vi "fpga_RefCH Process (50Hz).vi"(0 "data in <?24.1>":fxp<+/-,24,1>, 5 "Channel number":u8, 7 "Reference index":u8, 9 "input data valid":bool, 12 "ready for output":bool) -> (4 "Filtered Ref data":fxp<+/-,24,3> format="%.22g", 10 "output valid":bool, 15 "Timed Out":bool)   [LabVIEW 2011, in "NI_EP_Resample_FPGA.lvlib"]
uses:
  <vilib>/addons/Electrical Power/PQ/Resampling/NI_EP_Resample_FPGA.lvlib
  <vilib>/rvi/DataTransferAndStorage/Container/Common/niFpgaContainerState.ctl
  <vilib>/rvi/DataTransferAndStorage/Container/Common/niFpgaDataTypeControl.ctl
  <vilib>/rvi/DataTransferAndStorage/Container/Common/niFpgaContainerImplementationControl.ctl
  <vilib>/rvi/DataTransferAndStorage/Container/Common/niFpgaContainerArbitrationOptionsControl.ctl
  <vilib>/rvi/DataTransferAndStorage/Container/Common/niFpgaTransferTypeControl.ctl
  <vilib>/rvi/DataTransferAndStorage/Container/Common/niFpgaContainerInitializationParameters.ctl
  <vilib>/rvi/Memory/Memory_Types/niFpgaMemoryInterfaceConfiguration.ctl
  <vilib>/rvi/FIFO/Fifo_Types/niFpgaFifoControlLogicControl.ctl
  <vilib>/rvi/DataTransferAndStorage/Container/Common/niFpgaContainerMetaDataKey.ctl
  <vilib>/rvi/DataTransferAndStorage/Container/Common/niFpgaContainerGetUniqueNameForEmu.vi
  <vilib>/rvi/DataTransferAndStorage/Container/Common/niFpgaContainerSetEmuInfo.vi
  <vilib>/rvi/eio/common/nirviEmuReportErrorAndStop.vi
  <vilib>/rvi/FIFO/Fifo_Resource/nirvififoEmulationSetSize.vi
  <vilib>/rvi/LocalResourceManager/LocalResourceManager.xnode
  <vilib>/rvi/DataTransferAndStorage/Container/XNode/niFpgaContainer.xnode
  <vilib>/rvi/FIFO/Fifo_Resource/nirvififoEmulationWrite.vi
  <vilib>/rvi/FIFO/Fifo_Resource/nirvififoEmulationRead.vi
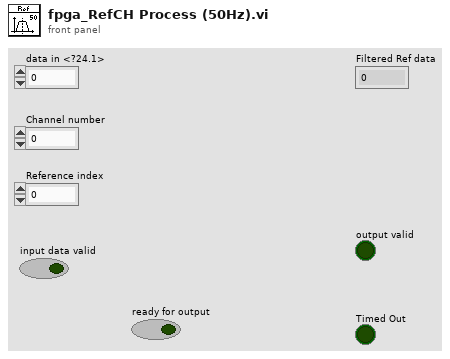
[diagram p1: front panel]
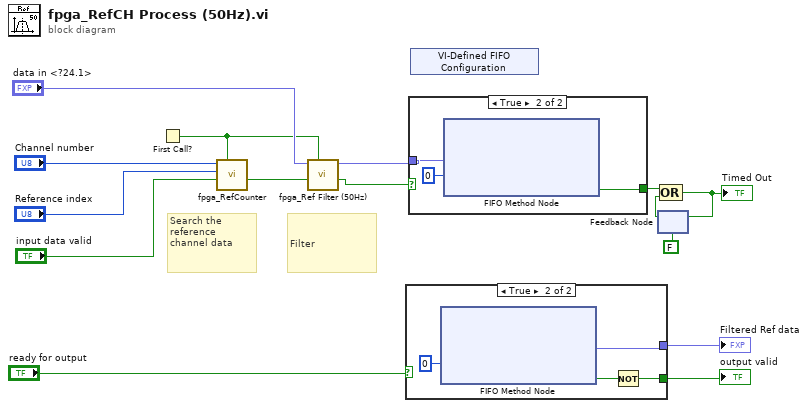
[diagram p0: block diagram]
diagram:
  # "Filter"
  # "Search the reference channel data"
  n1 = First Call?() -> (First Call?: T/F=w10:bool)
  n2 = call <vilib>:"fpga_RefCounter.vi"("reset"=w10, "input valid?"="input data valid", "Reference index"="Reference index", "NChan"="Channel number") -> ("Reference channel input valid"=w11:bool)  [unwired: 6 in, 1 out]
  n3 = call <vilib>:"fpga_Ref Filter (50Hz).vi"("reset"=w10, "input valid"=w11, "input data"="data in <?24.1>") -> ("output valid"=w2:bool, "output data <i24,3>"=w1:fxp<+/-,24,3>)  [unwired: 6 in, 1 out]
  n4 = case shown="True" "ready for output" {
    tunnel: [_ w18] -> w8
    tunnel: [_ w16] -> w9
    frame False {
    }
    frame True {
      n5 = xnode ("FIFO Method Node")("Timeout"=0) -> ("Element"=w18:fxp<+/-,24,3>, "Timed Out?"=w17:bool)  [unwired: 1 in, 1 out]
      n6 = Not(x=w17) -> (.not. x?=w16:bool)
    }
  }
  "output valid" <- w9
  "Filtered Ref data" <- w8
  n7 = case shown="True" w2 {
    tunnel: w1 -> [_ w22]
    tunnel: [_ w20] -> w4
    frame False {
    }
    frame True {
      n8 = xnode ("FIFO Method Node")("Element"=w22, "Timeout"=0) -> ("Timed Out?"=w20:bool)  [unwired: 1 in, 1 out]
    }
  }
  n9 = xnode "VI-Defined FIFO Configuration"() -> ()  [unwired: 1 out]
  n10 = feedback #1(FALSE) -> (w5:bool)
  n11 = Compound Arithmetic op=OR(w4, w5) -> (w3:bool)
  "Timed Out" <- w3
  n12 = feedback-in #1(w3) -> ()
